vi "Read Wrapback Data.vi"(2 "shared":refnum<class "niUSRP Rx Core v1 FPGA.lvclass">=refnum) -> (4 "I data":fxp<+/-,16,1>[](array[numeric]), 6 "Q data":fxp<+/-,16,1>[](array[numeric]))   [LabVIEW 2023, in "niUSRP Rx Core v1 FPGA.lvclass"]
doc: "this VI is used to wrap data from Generation output to Acquisition input."
uses:
  <instrlib>/niUSRP/Reference FPGA/Rx Core/niUSRP Rx Core v1 FPGA.lvclass
  <vilib>/rvi/DataTransferAndStorage/Container/XNode/niFpgaContainer.xnode
  <vilib>/rvi/DataTransferAndStorage/Register/Emulation/niFpgaRegisterEmulationRefIn.vi
  <instrlib>/niVST/Reference FPGA/FPGA/niUSRP Rx Core v1 FPGA/niUSRP Rx Core v1 FPGA.lvclass
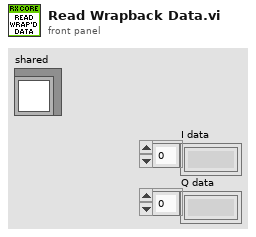
[diagram p1: front panel]
types:
  T1 = typedef "niVST Shared Registers v1 FPGA.lvclass/Shared Registers.ctl" = cluster{"wrapback data":refnum<k21>, "status.gen.generating":refnum<k21>, "status.gen.waiting for trigger":refnum<k21>, "status.acq.in progress":refnum<k21>, "status.acq.waiting for trigger":refnum<k21>}
  T2 = cluster{"I data":fxp<+/-,16,1>[], "Q data":fxp<+/-,16,1>[]}
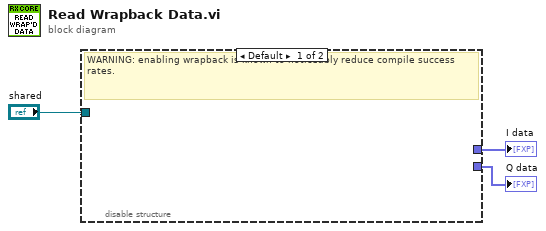
[diagram p0: block diagram]
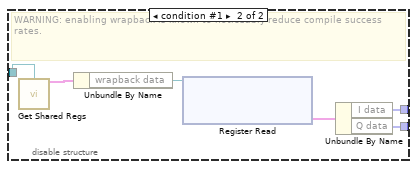
[diagram p2: hidden frame]
diagram:
  n1 = disable-structure shown="Default" {
    disable-tunnel: [_ w7] -> w3
    disable-tunnel: [_ w6] -> w2
    disable-tunnel: "shared" -> [_ w4]
    frame condition #0 (active) {
      # "WARNING: enabling wrapback is known to noticeably reduce compile success rates."
    }
    frame condition #1 {
      # "WARNING: enabling wrapback is known to noticeably reduce compile success rates."
      n2 = call-dynamic "Get Shared Regs.vi"("shared"=w4) -> ("shared regs"=w5:T1)  [unwired: 14 in]
      n3 = Unbundle By Name(w5) -> ("wrapback data"=w9:refnum<k21>)
      n4 = xnode "Register Read"("Register In"=w9) -> ("Data"=w8:T2)  [unwired: 1 out]
      n5 = Unbundle By Name(w8) -> ("I data"=w7:fxp<+/-,16,1>[], "Q data"=w6:fxp<+/-,16,1>[])
    }
  }
  "I data" <- w3
  "Q data" <- w2
